vi "ReScale Coeff 2D.vi"(6 "Gauss":bool, 7 "A":dbl=0.001, 9 "amplitude":dbl=1.0, 10 "Width":dbl=1.0, 11 "Array in":dbl[][](array[numeric])) -> (3 "Array out":dbl[][](array[numeric]))   [LabVIEW 2023]
uses:
  <vilib>/Analysis/1siggen.llb/Ramp Pattern by Samples.vi
  <vilib>/Analysis/1siggen.llb/General Gaussian Monopulse.vi
  <vilib>/Analysis/NI_AALBase.lvlib
panel:
  out "Ramp":dbl[](graph)
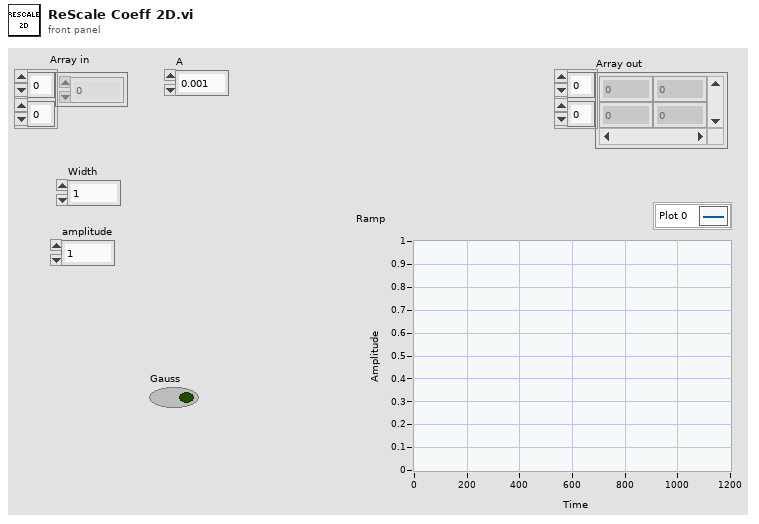
[diagram p1: front panel]
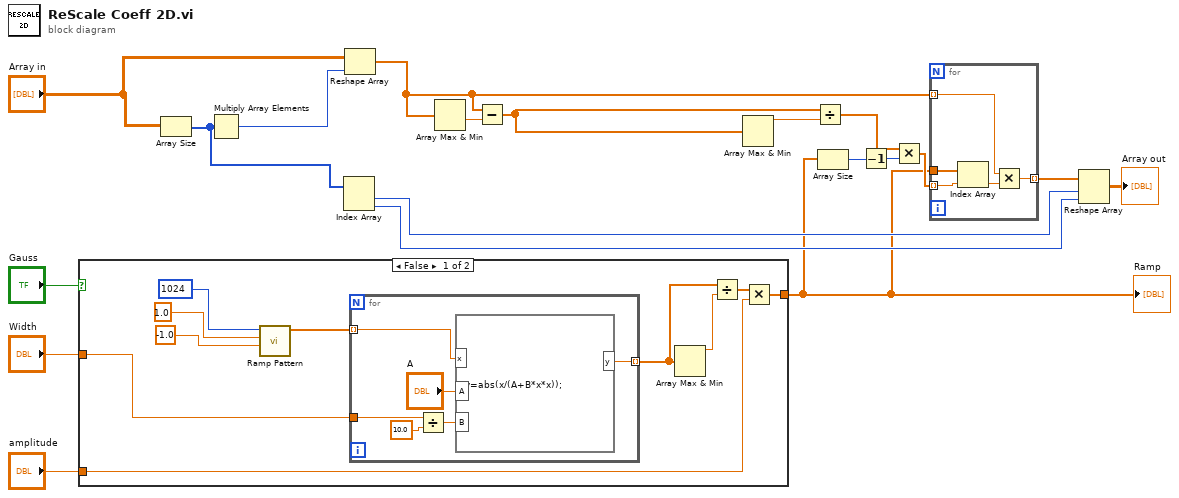
[diagram p0: block diagram]
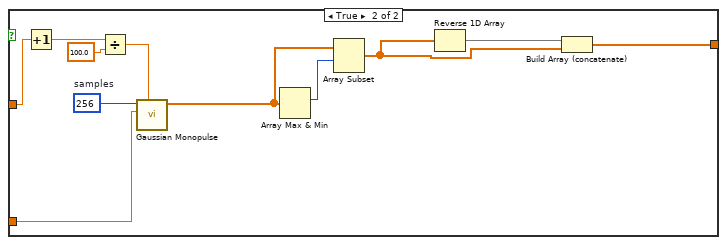
[diagram p2: hidden frame]
diagram:
  n1 = case shown="False" "Gauss" {
    tunnel: "amplitude" -> [w20 w46]
    tunnel: "Width" -> [w21 w37]
    tunnel: [w25 w36] -> w1
    frame False {
      n2 = call-poly <vilib>:"Ramp Pattern.vi"("start"=-1.0, "end"=1.0, "samples"=1024) -> ("Ramp Pattern"=w26:dbl[])  [unwired: 7 in, 1 out]
      n3 = for {
        tunnel: w26 -> [w35] mode=indexing
        tunnel: [w34] -> w24 mode=indexing
        tunnel: w21 -> [w32]
        n4 = Divide(x=w32, y=10.0) -> (x/y=w30:dbl)
        n5 = formula code="y=abs(x/(A+B*x*x));"("x"=w35, "A"="A", "B"=w30) -> ("y"=w34:dbl)
      }
      n6 = Array Max & Min(array=w24) -> (max value=w22:dbl)  [unwired: 3 out]
      n7 = Divide(x=w24, y=w22) -> (x/y=w23:dbl[])
      n8 = Multiply(x=w23, y=w20) -> (x*y=w25:dbl[])
    }
    frame True {
      w38 = 256  # samples
      n9 = Increment(x=w37) -> (x+1=w45:dbl)
      n10 = Divide(x=w45, y=100.0) -> (x/y=w43:dbl)
      n11 = call <vilib>:"Gaussian Monopulse.vi"("center frequency (Hz)"=w43, "amplitude"=w46, "samples"=w38) -> ("Gaussian Monopulse"=w39:dbl[])  [unwired: 7 in, 1 out]
      n12 = Array Max & Min(array=w39) -> (max index (indices)=w40:i32)  [unwired: 3 out]
      n13 = Array Subset(array=w39, index=w40) -> (w42:dbl[])  [unwired: 1 in]
      n14 = Reverse 1D Array(array=w42) -> (reversed array=w41:dbl[])
      n15 = Build Array (concatenate)(w41, w42) -> (w36:dbl[])
    }
  }
  "Ramp" <- w1
  n16 = Array Size(array="Array in") -> (size(s)=w6:i32[])
  n17 = Multiply Array Elements(1:w6) -> (0:w9:i32)
  n18 = Index Array(array=w6) -> (element #1=w5:i32, element #2=w4:i32)  [unwired: 2 in]
  n19 = Reshape Array("Array in", w9) -> (w8:dbl[])
  n20 = Array Max & Min(array=w8) -> (min value=w14:dbl)  [unwired: 3 out]
  n21 = Subtract(x=w8, y=w14) -> (x-y=w15:dbl[])
  n22 = Array Max & Min(array=w15) -> (max value=w16:dbl)  [unwired: 3 out]
  n23 = Divide(x=w15, y=w16) -> (x/y=w17:dbl[])
  n24 = Array Size(array=w1) -> (size(s)=w18:i32)
  n25 = Decrement(x=w18) -> (x-1=w2:i32)
  n26 = Multiply(x=w17, y=w2) -> (x*y=w19:dbl[])
  n27 = for {
    tunnel: w8 -> [w49] mode=indexing
    tunnel: w19 -> [w50] mode=indexing
    tunnel: w1 -> [w51]
    tunnel: [w47] -> w7 mode=indexing
    n28 = Index Array(array=w51, index=w50) -> (element=w48:dbl)
    n29 = Multiply(x=w49, y=w48) -> (x*y=w47:dbl)
  }
  n30 = Reshape Array(w7, w5, w4) -> (→"Array out":dbl[][])
